vi "GetFluidData (SubVI).vi"(8 "error in (no error)":errorcluster, 10 "Node":u8, 11 "VISA Refnum in":refnum<visa-resource-name>) -> (0 "error out":errorcluster, 3 "Fluid Data":T1)   [LabVIEW 2015]
uses:
  TypeDefs/FluidData.ctl
  <instrlib>/Bronkhorst FLOW-BUS/Bronkhorst FLOW-BUS.lvlib
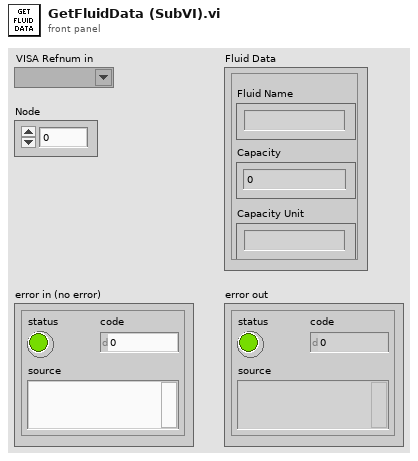
[diagram p1: front panel]
types:
  T1 = typedef "FluidData.ctl" = cluster{"Fluid Name":string, "Capacity":sgl, "Capacity Unit":string}
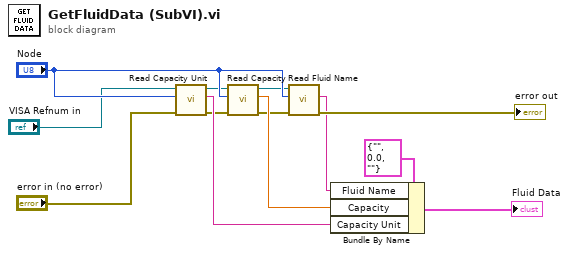
[diagram p0: block diagram]
diagram:
  n1 = call <instrlib>:"Read Capacity Unit.vi"("error in (no error)"="error in (no error)", "Node (3)"="Node", "VISA resource name"="VISA Refnum in") -> ("error out"=w3:errorcluster, "Capacity Unit"=w12:string, "VISA resource name out"=w4:refnum<visa-resource-name>)  [unwired: 6 in]
  n2 = call <instrlib>:"Read Capacity.vi"("error in (no error)"=w3, "Node (3)"="Node", "VISA resource name"=w4) -> ("error out"=w6:errorcluster, "Capacity"=w11:sgl, "VISA resource name out"=w5:refnum<visa-resource-name>)  [unwired: 6 in]
  n3 = call <instrlib>:"Read Fluid Name.vi"("error in (no error)"=w6, "Node (3)"="Node", "VISA resource name"=w5) -> ("error out"=→"error out":errorcluster, "Fluid Name"=w10:string)  [unwired: 6 in, 1 out]
  n4 = Bundle By Name(cluster=T1 {"Fluid Name"="", "Capacity"=0.0, "Capacity Unit"=""} ("Fluid Data"), "Fluid Name"=w10, "Capacity"=w11, "Capacity Unit"=w12) -> (→"Fluid Data":T1)
